vi "Sharp.vi"() -> ()   [LabVIEW 2018]
panel:
  out "Sharp IR Distance":dbl
  out "Raw Data":dbl
  in  "stop":bool
  out "error out":errorcluster
  in  "error in (no error)":errorcluster
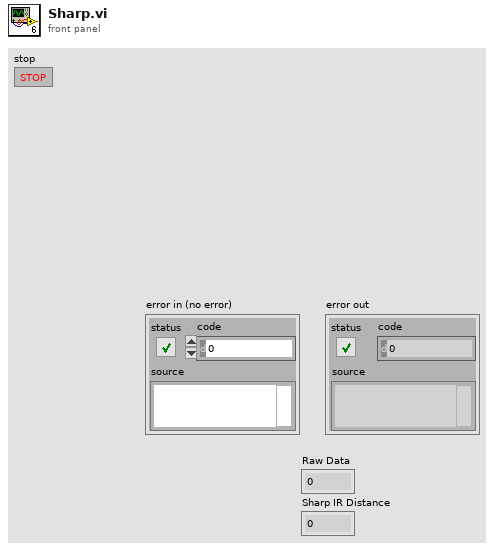
[diagram p1: front panel]
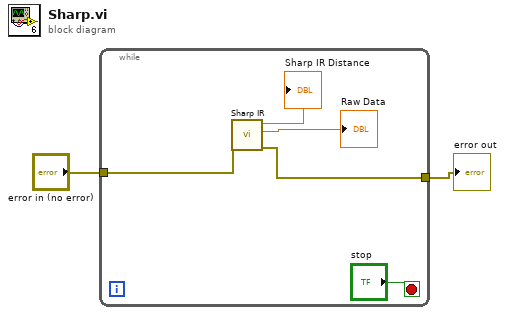
[diagram p0: block diagram]
diagram:
  n1 = while {
    tunnel: "error in (no error)" -> [w6]
    tunnel: [w5] -> w1
    stop <- "stop" stop-if-true
    n2 = call <vilib>:"Sharp IR.vi"("error in (no error)"=w6) -> ("error out"=w5:errorcluster, "Raw Data"=→"Raw Data":dbl, "Sharp IR Distance"=→"Sharp IR Distance":dbl)  [unwired: 8 in]
  }
  "error out" <- w1
